vi "S4GUI.vi"() -> ()   [LabVIEW 2018] (continued)
      tunnel: "Input Cluster" -> [_ _ _ _ _ _ _ _ _ _ _ _ _ _ _ _ w2328 w2364 _ _ _ _ _ _ _ _ _ _ _ _ _ _ _ _ _ _ _ _ _ _ _ _ _ _ _ _ _ _ _ _ _ _ _ _ _ _ _ _ _ _ _ _ _ _ _ _ _ _ _ _ _ _ _ _ _ _ _ _ _ _ _ _ _ _ _ _ _ _ _ _ _ _ _ _ _ _ _ _ _ _ _ _ _ _ _ _ _ _ _]
      tunnel: w60 -> [_ _ _ _ _ _ _ _ _ _ _ _ _ _ _ _ _ _ _ _ _ _ w3202 _ _ _ w4393 w4574 w4763 w4947 _ _ w5157 w5348 w5470 w5593 w5719 _ _ _ _ _ _ _ _ _ _ _ _ _ _ _ _ _ _ _ _ _ _ _ _ _ _ _ _ _ _ _ _ _ _ _ _ _ _ _ _ _ _ _ _ _ _ _ _ _ _ _ _ _ _ _ _ _ _ _ _ _ _ _ _ _ _ _ _ _ _ _ _]
      tunnel: w59 -> [_ _ _ _ _ _ _ _ _ _ _ _ _ _ _ _ _ _ _ _ _ _ w3201 _ _ _ _ w4577 w4766 w4950 _ _ w5161 w5347 w5469 w5594 w5718 _ _ _ _ _ _ _ _ _ _ _ _ _ _ _ _ _ _ _ _ _ _ _ _ _ _ _ _ _ _ _ _ _ _ _ _ _ _ _ _ _ _ _ _ _ _ _ _ _ _ _ _ _ _ _ _ _ _ _ _ _ _ _ _ _ _ _ _ _ _ _ _]
      tunnel: "Observer" -> [_ _ _ _ _ _ _ _ _ _ _ _ _ _ _ _ _ _ _ _ _ _ w3200 _ _ _ w4394 w4575 w4764 _ _ _ w5158 w5346 w5468 w5592 w5717 _ _ _ _ _ _ _ _ _ _ _ _ _ _ _ _ _ _ _ _ _ _ _ _ _ _ _ _ _ _ _ _ _ _ _ _ _ _ _ _ _ _ _ _ _ _ _ _ _ _ _ _ _ _ _ _ _ _ _ _ _ _ _ _ _ _ _ _ _ _ _ _]
      event Timeout {
        # "Obtém os valores de status dos\ndispositivos de cada servidor para\napresentar nos indicadores da GUI."
        # "Trata as tarefas individuais de \ncada servidor (ACS1,...,ACS4, \nICS, TCS, SyncBox)"
        # "Determina a sequência de\ntarefas dos servidores\npara uma observação, de \nacordo com o modo de \noperação (disparado com \nos botões START)"
        # "execução dos botões\n no modo sincrono."
        # "execução dos botões\n no modo assincrono."
        # "Instrument States.<device> State\n\n0: nao fez INIT e está parado (mode = IDLE ou WAITING\n                                                    contdition = default)\n1: nao fez INIT e está movendo (mode = IDLE ou WAITING\n                                                    contdition = BUSY)\n\n2: fez INIT e está parado (mode = default)\n                                            condition = READY)\n3: fez INIT e está movendo (mode = default)\n                                            condition = BUSY)"
        n76 = event-data() -> ()  [unwired: 1 in, 2 out]
        n77 = disable-structure shown="Enabled" {
          disable-tunnel: w137 -> [w145 w147]
          disable-tunnel: w136 -> [w144 w146]
          disable-tunnel: [w142 w146] -> w125
          disable-tunnel: [w141 w147] -> w124
          frame Disabled {
            n78 = call "Elapsed Time"() -> ("Time has Elapsed"=w140:bool)  [unwired: 12 in, 7 out]
            n79 = call "Elapsed Time3"() -> ("Time has Elapsed"=w143:bool)  [unwired: 12 in, 7 out]
            n80 = call "Write Status_timeout.vi"("error in (no error)"=w144, "TCS_timeout"=w143, "Status_timeout"=w140, "S4ACS_GUI in"=w145) -> ("error out"=w142:errorcluster, "S4ACS_GUI out"=w141:refnum<class "S4GUI.lvclass">)  [unwired: 6 in]
          }
          frame Enabled {
          }
        }
        n81 = call-dynamic "HandlePauseAsync.vi"("error in (no error)"=w125, "S4GUI in"=w124) -> ("error out"=w121:errorcluster, "S4GUI out"=w123:refnum<class "S4GUI.lvclass">)  [unwired: 8 in]
        n82 = call-dynamic "HandleStopAsync.vi"("error in (no error)"=w121, "S4GUI in"=w123) -> ("error out"=w120:errorcluster, "S4GUI out"=w122:refnum<class "S4GUI.lvclass">)  [unwired: 8 in]
        n83 = call-dynamic "HandleAbortAsync.vi"("error in (no error)"=w120, "S4GUI in"=w122) -> ("error out"=w114:errorcluster, "S4GUI out"=w115:refnum<class "S4GUI.lvclass">)  [unwired: 8 in]
        n84 = call-dynamic "HandlePauseSync.vi"("error in (no error)"=w114, "S4GUI in"=w115) -> ("error out"=w113:errorcluster, "S4GUI out"=w112:refnum<class "S4GUI.lvclass">)  [unwired: 8 in]
        n85 = call-dynamic "HandleStopSync.vi"("error in (no error)"=w113, "S4GUI in"=w112) -> ("error out"=w117:errorcluster, "S4GUI out"=w119:refnum<class "S4GUI.lvclass">)  [unwired: 8 in]
        n86 = call-dynamic "HandleAbortSync.vi"("error in (no error)"=w117, "S4GUI in"=w119) -> ("error out"=w116:errorcluster, "S4GUI out"=w118:refnum<class "S4GUI.lvclass">)  [unwired: 8 in]
        n87 = call-dynamic "HandleObservation.vi"("error in (no error)"=w116, "S4ACS_GUI in"=w118) -> ("error out"=w130:errorcluster, "S4ACS_GUI out"=w131:refnum<class "S4GUI.lvclass">)  [unwired: 8 in]
        n88 = call-dynamic "HandleServers.vi"("error in (no error)"=w130, "S4ACS_GUI in"=w131) -> ("error out"=w139:errorcluster, "S4ACS_GUI out"=w138:refnum<class "S4GUI.lvclass">)  [unwired: 8 in]
        n89 = call-dynamic "GetStatus.vi"("error in (no error)"=w139, "S4ACS_GUI in"=w138) -> ("error out"=w127:errorcluster, "output cluster"=w132:T9, "Cluster Disable"=w129:T10, "S4ACS_GUI out"=w128:refnum<class "S4GUI.lvclass">)  [unwired: 6 in]
        n90 = call "Read cfg file.vi"("error in (no error)"=w127, "S4ACS_GUI in"=w128) -> ("error out"=w109:errorcluster, "cfg file"=w126:string, "S4ACS_GUI out"=w110:refnum<class "S4GUI.lvclass">)  [unwired: 7 in]
        n91 = call "Elapsed Time2"() -> ("Time has Elapsed"=w111:bool)  [unwired: 12 in, 7 out]
        n92 = case shown="True" w111 {
          selector: w111 -> [_ w175]
          tunnel: w132 -> [_ w178]
          tunnel: w129 -> [_ w177]
          tunnel: w126 -> [_ w176]
          tunnel: w110 -> [w149 w172]
          tunnel: w109 -> [w148 w171]
          tunnel: [w149 w169] -> w108
          tunnel: [w148 w166] -> w107
          frame False {
          }
          frame True {
            # "MODE:\nF -> photometric\nT -> polarimetric"
            n93 = stacked-sequence {
              tunnel: w178 -> [w271 w272 w274 w276 w283 w313 w317 w466 w566 w805 _ _ _ _ _ w995 w1155 w1288 w1421]
              tunnel: [_ _ _ _ _ _ _ w464 _ _ _ _ _ _ _ _ _ _ _] -> w150
              tunnel: w177 -> [_ _ _ _ _ _ _ _ _ _ w828 w875 w887 w899 w911 _ _ _ _]
              tunnel: w175 -> [_ _ _ _ _ _ w314 _ w561 _ _ _ _ _ _ _ _ _ _]
              tunnel: w176 -> [_ _ _ _ _ _ _ _ _ _ _ _ _ _ _ w990 _ _ _]
              frame #0 {
                w233 = u32 240 ("Tab Control Pane Dimension:Width")
                w234 = u32 300 ("Tab Control Pane Dimension:Height")
                n94 = Unbundle By Name(w271) -> ("TCSPD_connection"=→"TCSPD":bool, "TCS extended"=w268:string)
                n95 = Match Pattern(string=w268, regular expression="RA=") -> (after substring=w264:string)  [unwired: 1 in, 3 out]
                n96 = Match Pattern(string=w264, regular expression="DEC=") -> (before substring=→"RA":string, after substring=w263:string)  [unwired: 1 in, 2 out]
                n97 = Match Pattern(string=w263, regular expression="EQUINOX=") -> (before substring=→"DEC":string, after substring=w262:string)  [unwired: 1 in, 2 out]
                n98 = Match Pattern(string=w262, regular expression="AIRMASS=") -> (after substring=w258:string)  [unwired: 1 in, 3 out]
                n99 = Match Pattern(string=w258, regular expression="TCSHA=") -> (before substring=→"Air Mass":string, after substring=w257:string)  [unwired: 1 in, 2 out]
                n100 = Match Pattern(string=w257, regular expression="TCSDATE=") -> (before substring=→"Hour Angle":string, after substring=w255:string)  [unwired: 1 in, 2 out]
                n101 = Match Pattern(string=w255, regular expression="TELFOCUS=") -> (before substring=→"Date":string, after substring=w251:string)  [unwired: 1 in, 2 out]
                n102 = Match Pattern(string=w251, regular expression="EXTTEMP=") -> (before substring=→"Telescope Focus":string, after substring=w250:string)  [unwired: 1 in, 2 out]
                n103 = Match Pattern(string=w250, regular expression="PRESSURE=") -> (before substring=→"Outside Temp":string, after substring=w249:string)  [unwired: 1 in, 2 out]
                n104 = property on="Tab CH2" class="TabCtl (strict)"("PaneHeight"=w234, "PaneWidth"=w233) -> ()  [unwired: 2 in, 2 out]
                n105 = property on="Tab CH1" class="TabCtl (strict)"("PaneHeight"=w234, "PaneWidth"=w233) -> ()  [unwired: 2 in, 2 out]
                n106 = property on="Tab CH3" class="TabCtl (strict)"("PaneHeight"=w234, "PaneWidth"=w233) -> ()  [unwired: 2 in, 2 out]
                n107 = Match Pattern(string=w249, regular expression="HUMIDITY=") -> (before substring=→"Pressure":string, after substring=w238:string)  [unwired: 1 in, 2 out]
                n108 = property on="Tab CH4" class="TabCtl (strict)"("PaneHeight"=w234, "PaneWidth"=w233) -> ()  [unwired: 2 in, 2 out]
                n109 = Match Pattern(string=w238, regular expression="JD=") -> (before substring=→"Humidity":string, after substring=w239:string)  [unwired: 1 in, 2 out]
                n110 = Match Pattern(string=w239, regular expression="SD=") -> (before substring=→"Julian Date":string, after substring=→"Sideral Time":string)  [unwired: 1 in, 2 out]
              }
              frame #1 {
                n111 = Unbundle By Name(w272) -> ()  [unwired: 1 out]
              }
              frame #2 {
                n112 = Unbundle By Name(w274) -> ("Trigger Mode Status"=→"String":string)
              }
              frame #3 {
                n113 = Unbundle By Name(w276) -> ("Trigger General Status"=→"String 2":string)
              }
              frame #4 {
                n114 = Unbundle By Name(w283) -> ("Instrument Status"=w282:T11, "Instrument States.WPROT State"=w281:i32, "Instrument Pos Names.WPROT posname"=w280:string, "Instrument Pos Names.WPSEL posname"=w279:string, "Instrument Pos Names.CALW posname"=w278:string, "Instrument Pos Names.ASEL posname"=w277:string)
                n115 = stacked-sequence {
                  tunnel: w282 -> [w290 w293 w296 w298 w300 w303 w306 w308 w310]
                  tunnel: w281 -> [w286 _ _ _ _ _ _ _ _]
                  tunnel: w280 -> [_ w291 _ _ _ _ _ _ _]
                  tunnel: w279 -> [_ _ w294 _ _ _ _ _ _]
                  tunnel: w278 -> [_ _ _ _ _ w301 _ _ _]
                  tunnel: w277 -> [_ _ _ _ _ _ w304 _ _]
                  frame #0 {
                    # "Pisca quando BUSY"
                    n116 = Unbundle By Name(w290) -> ("WPROT pos"=w287:dbl)
                    "WaveplatePos 2" <- w287
                    n117 = Equal?(x=w286, y=3) -> (x = y?=w284:bool)
                    n118 = property on="WaveplatePos 2" class="DigNum (strict)"("Blinking"=w284) -> ()  [unwired: 2 in, 2 out]
                    n119 = Number To Fractional String(number=w287, precision (6)=i16 1) -> (F-format string=→"Angle":string)  [unwired: 2 in]
                  }
                  frame #1 {
                    n120 = Unbundle By Name(w293) -> ("WPROT pos"=→"Position WPROT":dbl)
                    "PosName WPROT" <- w291
                  }
                  frame #2 {
                    n121 = Unbundle By Name(w296) -> ("WPSEL pos"=→"Position WPSEL":dbl)
                    "PosName WPSEL" <- w294
                  }
                  frame #3 {
                    n122 = Unbundle By Name(w298) -> ("GMIR pos"=→"Position GMIR":dbl)
                  }
                  frame #4 {
                    n123 = Unbundle By Name(w300) -> ("GFOC pos"=→"Position GFOC":dbl)
                  }
                  frame #5 {
                    n124 = Unbundle By Name(w303) -> ("CALW pos"=→"Position CALW":dbl)
                    "PosName CALW" <- w301
                  }
                  frame #6 {
                    n125 = Unbundle By Name(w306) -> ("ASEL pos"=→"PosName ASEL":dbl)
                    "PosName ASEL" <- w304
                  }
                  frame #7 {
                    n126 = Unbundle By Name(w308) -> ("connection"=→"S4ICSoft":bool)
                  }
                  frame #8 {
                    n127 = Unbundle By Name(w310) -> ("String Status"=→"Status":string)
                  }
                }
              }
              frame #5 {
                n128 = Unbundle By Name(w313) -> ("Sync Box State"=→"Current State":i32, "Trigger_connection"=→"Sync Box" →"LedExtSync":bool)
              }
              frame #6 {
                n129 = Unbundle By Name(w317) -> ("Instrument States"=w316:T12, "Instrument Pos Names"=w315:T13)
                n130 = stacked-sequence {
                  tunnel: w316 -> [w326 w352 w371 w410 w439 w453]
                  tunnel: w315 -> [w322 _ w369 w406 _ _]
                  tunnel: w314 -> [w320 _ w363 w403 _ _]
                  frame #0 {
                    # "WPSEL"
                    n131 = Unbundle By Name(w322) -> ("WPSEL posname"=w318:string)
                    n132 = Unbundle By Name(w326) -> ("WPSEL State"=w325:i32)
                    n133 = local read "WPSEL Status"() -> (w321:bool)
                    n134 = case shown="2" w325 {
                      tunnel: [cluster{u32, u32}[] [{9868950, 9868950}, {9868950, 9868950}] ("Colors [4]") cluster{u32, u32}[] [{9868950, 9868950}, {9868950, 9868950}] ("Colors [4]") cluster{u32, u32}[] [{16318208, 16318208}, {16318208, 16318208}] ("Colors [4]") cluster{u32, u32}[] [{6618880, 2424594}, {6618880, 2424594}] ("Colors [4]") w341] -> w324
                      tunnel: [FALSE ("WPROT Status") FALSE ("WPROT Status") TRUE ("WPROT Status") FALSE ("WPROT Status") w343] -> w323
                      tunnel: w321 -> [_ _ _ _ w342]
                      tunnel: w320 -> [_ _ _ _ w340]
                      tunnel: ["" "" "" w336 ""] -> w319
                      tunnel: w318 -> [_ _ _ w336 _]
                      frame Default {
                      }
                      frame 0 {
                      }
                      frame 1 {
                      }
                      frame 2 {
                      }
                      frame 3 {
                        n135 = case shown="True" w342 {
                          tunnel: [cluster{u32, u32}[] [{7563008, 7563008}, {7563008, 7563008}] ("Colors [4]") cluster{u32, u32}[] [{16318208, 16318208}, {16318208, 16318208}] ("Colors [4]")] -> w341
                          frame False {
                          }
                          frame True {
                          }
                        }
                        n136 = case shown="True" w340 {
                          tunnel: [w344 w346] -> w343
                          tunnel: w342 -> [w344 w345]
                          frame False {
                          }
                          frame True {
                            n137 = Not(x=w345) -> (.not. x?=w346:bool)
                          }
                        }
                      }
                    }
                    "WPSEL Status" <- w323
                    "Waveplate" <- w323
                    n138 = property on="Waveplate" class="Bool (strict)"("Colors [4]"=w324, "BoolText.Text"=w319) -> ()  [unwired: 2 in, 2 out]
                    n139 = property on="WPSEL Status" class="Bool (strict)"("Colors [4]"=w324) -> ()  [unwired: 2 in, 2 out]
                  }
                  frame #1 {
                    # "WPROT"
                    n140 = Unbundle By Name(w352) -> ("WPROT State"=w351:i32)
                    n141 = case shown="2" w351 {
                      tunnel: [cluster{u32, u32}[] [{9868950, 9868950}, {9868950, 9868950}] ("Colors [4]") cluster{u32, u32}[] [{9868950, 9868950}, {9868950, 9868950}] ("Colors [4]") cluster{u32, u32}[] [{16318208, 16318208}, {16318208, 16318208}] ("Colors [4]") cluster{u32, u32}[] [{6618880, 6618880}, {6618880, 6618880}] ("Colors [4]") cluster{u32, u32}[] [{16318208, 16318208}, {16318208, 16318208}] ("Colors [4]")] -> w350
                      tunnel: [FALSE ("WPROT Status") FALSE ("WPROT Status") TRUE ("WPROT Status") FALSE ("WPROT Status") TRUE ("WPROT Status")] -> w349
                      frame Default {
                      }
                      frame 0 {
                      }
                      frame 1 {
                      }
                      frame 2 {
                      }
                      frame 3 {
                      }
                    }
                    "WPROT Status" <- w349
                    n142 = property on="WPROT Status" class="Bool (strict)"("Colors [4]"=w350) -> ()  [unwired: 2 in, 2 out]
                  }
                  frame #2 {
                    # "CALW"
                    n143 = Unbundle By Name(w371) -> ("CALW State"=w370:i32)
                    n144 = Unbundle By Name(w369) -> ("CALW posname"=w368:string)
                    n145 = local read "CALW Status"() -> (w364:bool)
                    n146 = case shown="Default" w370 {
                      tunnel: [cluster{u32, u32}[] [{9868950, 9868950}, {9868950, 9868950}] ("Colors [4]") cluster{u32, u32}[] [{9868950, 9868950}, {9868950, 9868950}] ("Colors [4]") cluster{u32, u32}[] [{16318208, 16318208}, {16318208, 16318208}] ("Colors [4]") cluster{u32, u32}[] [{6618880, 6618880}, {6618880, 6618880}] ("Colors [4]") w392] -> w365
                      tunnel: [FALSE ("WPROT Status") FALSE ("WPROT Status") TRUE ("WPROT Status") FALSE ("WPROT Status") w394] -> w367
                      tunnel: w368 -> [_ _ _ w382 _]
                      tunnel: ["" "" "" w381 ""] -> w366
                      tunnel: w364 -> [_ _ _ _ w393]
                      tunnel: w363 -> [_ _ _ _ w391]
                      frame Default {
                      }
                      frame 0 {
                      }
                      frame 1 {
                      }
                      frame 2 {
                        n147 = case shown="\"SHUTTER\"" w382 {
                          tunnel: ["" "DEPOL" "POL" "OFF" "PIN" "SHT"] -> w381
                          frame Default {
                          }
                          frame "DEPOLARIZER" {
                          }
                          frame "POLARIZER" {
                          }
                          frame "OFF" {
                          }
                          frame "PINHOLE" {
                          }
                          frame "SHUTTER" {
                          }
                        }
                      }
                      frame 3 {
                        n148 = case shown="False" w393 {
                          tunnel: [cluster{u32, u32}[] [{7563008, 7563008}, {7563008, 7563008}] ("Colors [4]") cluster{u32, u32}[] [{16318208, 16318208}, {16318208, 16318208}] ("Colors [4]")] -> w392
                          frame False {
                          }
                          frame True {
                          }
                        }
                        n149 = case shown="True" w391 {
                          tunnel: [w396 w398] -> w394
                          tunnel: w393 -> [w396 w397]
                          frame False {
                          }
                          frame True {
                            n150 = Not(x=w397) -> (.not. x?=w398:bool)
                          }
                        }
                      }
                    }
                    "CALW Status" <- w367
                    "PCS" <- w367
                    n151 = property on="CALW Status" class="Bool (strict)"("Colors [4]"=w365) -> ()  [unwired: 2 in, 2 out]
                    n152 = property on="PCS" class="Bool (strict)"("Colors [4]"=w365, "BoolText.Text"=w366) -> ()  [unwired: 2 in, 2 out]
                  }
                  frame #3 {
                    # "ASEL"
                    n153 = Unbundle By Name(w410) -> ("ASEL State"=w409:i32)
                    n154 = Unbundle By Name(w406) -> ("ASEL posname"=w402:string)
                    n155 = local read "ASEL Status"() -> (w404:bool)
                    n156 = case shown="Default" w402 {
                      selector: w402 -> [w411 _ _]
                      tunnel: [w411 "OFF" ("y") "ON" ("y")] -> w401
                      frame Default {
                      }
                      frame "OFF" {
                      }
                      frame "ON" {
                      }
                    }
                    n157 = case shown="2" w409 {
                      tunnel: [cluster{u32, u32}[] [{9868950, 9868950}, {9868950, 9868950}] ("Colors [4]") cluster{u32, u32}[] [{9868950, 9868950}, {9868950, 9868950}] ("Colors [4]") cluster{u32, u32}[] [{16318208, 16318208}, {16318208, 16318208}] ("Colors [4]") cluster{u32, u32}[] [{6618880, 6618880}, {6618880, 6618880}] ("Colors [4]") w430] -> w407
                      tunnel: [FALSE ("WPROT Status") FALSE ("WPROT Status") TRUE FALSE ("WPROT Status") w429] -> w408
                      tunnel: w401 -> [_ _ _ w424 _]
                      tunnel: ["" ("y") "" ("y") "" ("y") w424 "" ("y")] -> w405
                      tunnel: w404 -> [_ _ _ _ w427]
                      tunnel: w403 -> [_ _ _ _ w426]
                      frame Default {
                      }
                      frame 0 {
                      }
                      frame 1 {
                      }
                      frame 2 {
                      }
                      frame 3 {
                        n158 = case shown="True" w427 {
                          tunnel: [cluster{u32, u32}[] [{7563008, 7563008}, {7563008, 7563008}] ("Colors [4]") cluster{u32, u32}[] [{16318208, 16318208}, {16318208, 16318208}] ("Colors [4]")] -> w430
                          frame False {
                          }
                          frame True {
                          }
                        }
                        n159 = case shown="True" w426 {
                          tunnel: [w431 w433] -> w429
                          tunnel: w427 -> [w431 w432]
                          frame False {
                          }
                          frame True {
                            n160 = Not(x=w432) -> (.not. x?=w433:bool)
                          }
                        }
                      }
                    }
                    "ASEL Status" <- w408
                    "Analyzer" <- w408
                    n161 = property on="Analyzer" class="Bool (strict)"("Colors [4]"=w407, "BoolText.Text"=w405) -> ()  [unwired: 2 in, 2 out]
                    n162 = property on="ASEL Status" class="Bool (strict)"("Colors [4]"=w407) -> ()  [unwired: 2 in, 2 out]
                  }
                  frame #4 {
                    # "GMIR"
                    n163 = Unbundle By Name(w439) -> ("GMIR State"=w438:i32)
                    n164 = case shown="2" w438 {
                      tunnel: [cluster{u32, u32}[] [{9868950, 9868950}, {9868950, 9868950}] ("Colors [4]") cluster{u32, u32}[] [{9868950, 9868950}, {9868950, 9868950}] ("Colors [4]") cluster{u32, u32}[] [{16318208, 16318208}, {16318208, 16318208}] ("Colors [4]") cluster{u32, u32}[] [{6618880, 6618880}, {6618880, 6618880}] ("Colors [4]") cluster{u32, u32}[] [{16318208, 16318208}, {16318208, 16318208}] ("Colors [4]")] -> w437
                      tunnel: [FALSE ("WPROT Status") FALSE ("WPROT Status") TRUE ("WPROT Status") FALSE ("WPROT Status") TRUE ("WPROT Status")] -> w436
                      frame Default {
                      }
                      frame 0 {
                      }
                      frame 1 {
                      }
                      frame 2 {
                      }
                      frame 3 {
                      }
                    }
                    "GMIR Status" <- w436
                    n165 = property on="GMIR Status" class="Bool (strict)"("Colors [4]"=w437) -> ()  [unwired: 2 in, 2 out]
                  }
                  frame #5 {
                    # "GFOC"
                    n166 = Unbundle By Name(w453) -> ("GFOC State"=w452:i32)
                    n167 = case shown="0" w452 {
                      tunnel: [cluster{u32, u32}[] [{9868950, 9868950}, {9868950, 9868950}] ("Colors [4]") cluster{u32, u32}[] [{9868950, 9868950}, {9868950, 9868950}] ("Colors [4]") cluster{u32, u32}[] [{16318208, 16318208}, {16318208, 16318208}] ("Colors [4]") cluster{u32, u32}[] [{6618880, 6618880}, {6618880, 6618880}] ("Colors [4]") cluster{u32, u32}[] [{16318208, 16318208}, {16318208, 16318208}] ("Colors [4]")] -> w451
                      tunnel: [FALSE ("WPROT Status") FALSE ("WPROT Status") TRUE ("WPROT Status") FALSE ("WPROT Status") TRUE ("WPROT Status")] -> w450
                      frame Default {
                      }
                      frame 0 {
                      }
                      frame 1 {
                      }
                      frame 2 {
                      }
                      frame 3 {
                      }
                    }
                    "GFOC Status" <- w450
                    n168 = property on="GFOC Status" class="Bool (strict)"("Colors [4]"=w451) -> ()  [unwired: 2 in, 2 out]
                  }
                }
              }
              frame #7 {
                n169 = Unbundle By Name(w466) -> ("Instrument Pos Names"=w465:T13)
                n170 = stacked-sequence {
                  tunnel: w465 -> [w468 w485 w510 w536]
                  tunnel: [_ _ _ w537] -> w464
                  frame #0 {
                    n171 = Unbundle By Name(w468) -> ("WPSEL posname"=w467:string)
                    n172 = case shown="\"L/2\", \"L/4\", \"OFF\"" w467 {
                      selector: w467 -> [_ w469]
                      frame "False", Default {
                      }
                      frame "L/2", "L/4", "OFF" {
                        n173 = First Call?() -> (First Call?: T/F=w470:bool)
                        n174 = case shown="True" w470 {
                          tunnel: w469 -> [_ w471]
                          frame False {
                          }
                          frame True {
                            n175 = case shown="\"L/2\"" w471 {
                              frame "False", Default {
                              }
                              frame "L/2" {
                                w472 = u16 1 items=["OFF", "Lambda/2", "Lambda/4"] ("Lambda Selector")
                                n176 = property on="Lambda Selector" class="Ring (strict)"(error in=errorcluster {"status"=FALSE, "code"=0, "source"=""} ("error in (no error)"), "Value"=w472) -> (error out=w474:errorcluster)  [unwired: 1 in, 1 out]
                                n177 = property on="Lambda Selector" class="Ring (strict)"(error in=w474, "RingText.Text"="Lambda/2" ("Boolean Text.Text")) -> ()  [unwired: 1 in, 2 out]
                              }
                              frame "L/4" {
                                w476 = u16 2 items=["OFF", "Lambda/2", "Lambda/4"] ("Lambda Selector")
                                n178 = property on="Lambda Selector" class="Ring (strict)"(error in=errorcluster {"status"=FALSE, "code"=0, "source"=""} ("error in (no error)"), "Value"=w476) -> (error out=w478:errorcluster)  [unwired: 1 in, 1 out]
                                n179 = property on="Lambda Selector" class="Ring (strict)"(error in=w478, "RingText.Text"="Lambda/4" ("Boolean Text.Text")) -> ()  [unwired: 1 in, 2 out]
                              }
                              frame "OFF" {
                                w480 = u16 0 items=["OFF", "Lambda/2", "Lambda/4"] ("Lambda Selector")
                                n180 = property on="Lambda Selector" class="Ring (strict)"(error in=errorcluster {"status"=FALSE, "code"=0, "source"=""} ("error in (no error)"), "Value"=w480) -> (error out=w482:errorcluster)  [unwired: 1 in, 1 out]
                                n181 = property on="Lambda Selector" class="Ring (strict)"(error in=w482, "RingText.Text"="OFF" ("Boolean Text.Text")) -> ()  [unwired: 1 in, 2 out]
                              }
                            }
                          }
                        }
                      }
                    }
                  }
                  frame #1 {
                    n182 = Unbundle By Name(w485) -> ("CALW posname"=w484:string)
                    n183 = case shown="\"DEPOLARIZER\", \"OFF\", \"PINHOLE\", \"POLARIZER\", \"SHUTTER\"" w484 {
                      selector: w484 -> [_ w486]
                      frame "False", Default {
                      }
                      frame "DEPOLARIZER", "OFF", "PINHOLE", "POLARIZER", "SHUTTER" {
                        n184 = First Call?() -> (First Call?: T/F=w487:bool)
                        n185 = case shown="True" w487 {
                          tunnel: w486 -> [_ w488]
                          frame False {
                          }
                          frame True {
                            n186 = case shown="\"OFF\"" w488 {
                              frame "False", Default {
                              }
                              frame "POLARIZER" {
                                w489 = u16 1 items=["OFF", "POLARIZER", "PINHOLE", "SHUTTER", "DEPOLARIZER"] ("Calibrator Selector")
                                n187 = property on="Calibrator Selector" class="Ring (strict)"(error in=errorcluster {"status"=FALSE, "code"=0, "source"=""} ("error in (no error)"), "Value"=w489) -> (error out=w491:errorcluster)  [unwired: 1 in, 1 out]
                                n188 = property on="Calibrator Selector" class="Ring (strict)"(error in=w491, "RingText.Text"="POLARIZER" ("Boolean Text.Text")) -> ()  [unwired: 1 in, 2 out]
                              }
                              frame "DEPOLARIZER" {
                                w493 = u16 4 items=["OFF", "POLARIZER", "PINHOLE", "SHUTTER", "DEPOLARIZER"] ("Calibrator Selector")
                                n189 = property on="Calibrator Selector" class="Ring (strict)"(error in=errorcluster {"status"=FALSE, "code"=0, "source"=""} ("error in (no error)"), "Value"=w493) -> (error out=w495:errorcluster)  [unwired: 1 in, 1 out]
                                n190 = property on="Calibrator Selector" class="Ring (strict)"(error in=w495, "RingText.Text"="DEPOLARIZER" ("Boolean Text.Text")) -> ()  [unwired: 1 in, 2 out]
                              }
                              frame "PINHOLE" {
                                w497 = u16 2 items=["OFF", "POLARIZER", "PINHOLE", "SHUTTER", "DEPOLARIZER"] ("Calibrator Selector")
                                n191 = property on="Calibrator Selector" class="Ring (strict)"(error in=errorcluster {"status"=FALSE, "code"=0, "source"=""} ("error in (no error)"), "Value"=w497) -> (error out=w499:errorcluster)  [unwired: 1 in, 1 out]
                                n192 = property on="Calibrator Selector" class="Ring (strict)"(error in=w499, "RingText.Text"="PINHOLE" ("Boolean Text.Text")) -> ()  [unwired: 1 in, 2 out]
                              }
                              frame "SHUTTER" {
                                w501 = u16 3 items=["OFF", "POLARIZER", "PINHOLE", "SHUTTER", "DEPOLARIZER"] ("Calibrator Selector")
                                n193 = property on="Calibrator Selector" class="Ring (strict)"(error in=errorcluster {"status"=FALSE, "code"=0, "source"=""} ("error in (no error)"), "Value"=w501) -> (error out=w503:errorcluster)  [unwired: 1 in, 1 out]
                                n194 = property on="Calibrator Selector" class="Ring (strict)"(error in=w503, "RingText.Text"="SHUTTER" ("Boolean Text.Text")) -> ()  [unwired: 1 in, 2 out]
                              }
                              frame "OFF" {
                                w505 = u16 0 items=["OFF", "POLARIZER", "PINHOLE", "SHUTTER", "DEPOLARIZER"] ("Calibrator Selector")
                                n195 = property on="Calibrator Selector" class="Ring (strict)"(error in=errorcluster {"status"=FALSE, "code"=0, "source"=""} ("error in (no error)"), "Value"=w505) -> (error out=w507:errorcluster)  [unwired: 1 in, 1 out]
                                n196 = property on="Calibrator Selector" class="Ring (strict)"(error in=w507, "RingText.Text"="OFF" ("Boolean Text.Text")) -> ()  [unwired: 1 in, 2 out]
                              }
                            }
                          }
                        }
                      }
                    }
                  }
                  frame #2 {
                    n197 = Unbundle By Name(w510) -> ("WPROT posname"=w509:string)
                    "Name" <- w509
                    n198 = stacked-sequence {
                      tunnel: w509 -> [_ w512]
                      frame #0 {
                        w511 = FALSE
                        "ledP0" <- w511
                        "ledP1" <- w511
                        "ledP2" <- w511
                        "ledP3" <- w511
                        "ledP4" <- w511
                        "ledP5" <- w511
                        "ledP6" <- w511
                        "ledP7" <- w511
                        "ledP8" <- w511
                        "ledP9" <- w511
                        "ledP10" <- w511
                        "ledP11" <- w511
                        "ledP12" <- w511
                        "ledP13" <- w511
                        "ledP14" <- w511
                        "ledP15" <- w511
                      }
                      frame #1 {
                        n199 = case shown="\"WP15\"" w512 {
                          frame Default {
                          }
                          frame "WP1" {
                            n200 = local write "ledP0"(TRUE ("ledP0")) -> ()
                          }
                          frame "WP2" {
                            n201 = local write "ledP1"(TRUE ("ledP0")) -> ()
                          }
                          frame "WP3" {
                            n202 = local write "ledP2"(TRUE ("ledP0")) -> ()
                          }
                          frame "WP4" {
                            n203 = local write "ledP3"(TRUE ("ledP0")) -> ()
                          }
                          frame "WP5" {
                            n204 = local write "ledP4"(TRUE ("ledP0")) -> ()
                          }
                          frame "WP6" {
                            n205 = local write "ledP5"(TRUE ("ledP0")) -> ()
                          }
                          frame "WP7" {
                            n206 = local write "ledP6"(TRUE ("ledP0")) -> ()
                          }
                          frame "WP8" {
                            n207 = local write "ledP7"(TRUE ("ledP0")) -> ()
                          }
                          frame "WP9" {
                            n208 = local write "ledP8"(TRUE ("ledP0")) -> ()
                          }
                          frame "WP10" {
                            n209 = local write "ledP9"(TRUE ("ledP0")) -> ()
                          }
                          frame "WP11" {
                            n210 = local write "ledP10"(TRUE ("ledP0")) -> ()
                          }
                          frame "WP12" {
                            n211 = local write "ledP11"(TRUE ("ledP0")) -> ()
                          }
                          frame "WP13" {
                            n212 = local write "ledP12"(TRUE ("ledP0")) -> ()
                          }
                          frame "WP14" {
                            n213 = local write "ledP13"(TRUE ("ledP0")) -> ()
                          }
                          frame "WP15" {
                            n214 = local write "ledP14"(TRUE ("ledP0")) -> ()
                          }
                          frame "WP16" {
                            n215 = local write "ledP15"(TRUE ("ledP0")) -> ()
                          }
                        }
                      }
                    }
                  }
                  frame #3 {
                    w540 = "OFF" ("Boolean Text.Text")
                    # "Polarimetria:   ASEL = ON  &   (WPSEL =L/2 or L/4)\n\nFotometria:    ASEL=OFF & WPSEL = OFF & CALW = OFF"
                    n216 = Unbundle By Name(w536) -> ("ASEL posname"=w531:string, "WPSEL posname"=w533:string, "ASEL posname"=w532:string)
                    n217 = Unbundle By Name(w536) -> ("WPSEL posname"=w543:string, "CALW posname"=w544:string, "ASEL posname"=w538:string)
                    n218 = Equal?(x=w531, y="ON" ("Boolean Text.Text")) -> (x = y?=w534:bool)
                    n219 = case shown="True" w534 {
                      tunnel: w533 -> [w553 w558]
                      tunnel: w532 -> [w552 _]
                      tunnel: w531 -> [w549 _]
                      tunnel: [FALSE ("Polarimetric Mode") w555] -> w530
                      tunnel: [w545 FALSE ("Photometric Mode")] -> w529
                      frame False {
                        w548 = "OFF" ("Boolean Text.Text")
                        n220 = Equal?(x=w549, y=w548) -> (x = y?=w547:bool)
                        n221 = Equal?(x=w552, y=w548) -> (x = y?=w550:bool)
                        n222 = Equal?(x=w553, y=w548) -> (x = y?=w551:bool)
                        n223 = Compound Arithmetic op=AND(w547, w551, w550) -> (w545:bool)
                      }
                      frame True {
                        n224 = Equal?(x="L/2" ("Boolean Text.Text"), y=w558) -> (x = y?=w559:bool)
                        n225 = Equal?(x="L/4" ("Boolean Text.Text"), y=w558) -> (x = y?=w556:bool)
                        n226 = Or(x=w559, y=w556) -> (x .or. y?=w555:bool)
                      }
                    }
                    "Polarimetric Mode" <- w530
                    "Photometric Mode" <- w529
                    n227 = Equal?(x=w540, y=w543) -> (x = y?=w541:bool)
                    n228 = Equal?(x=w540, y=w544) -> (x = y?=w542:bool)
                    n229 = Equal?(x=w540, y=w538) -> (x = y?=w539:bool)
                    n230 = Compound Arithmetic op=AND(w541, w542, w539) -> (invert w537:bool)
                  }
                }
              }
              frame #8 {
                n231 = Unbundle By Name(w566) -> ("ChannelA_Status"=w565:T14, "ChannelB_Status"=w564:T14, "ChannelC_Status"=w562:T14, "ChannelD_Status"=w563:T14)
                n232 = stacked-sequence {
                  tunnel: w565 -> [w614 w662 w715 w791 _ _ _]
                  tunnel: w564 -> [w613 w660 w714 _ w794 _ _]
                  tunnel: w563 -> [w611 w657 w712 _ _ _ w802]
                  tunnel: w562 -> [w612 w658 w713 _ _ w798 _]
                  tunnel: w561 -> [_ _ w704 _ _ _ _]
                  frame #0 {
                    n233 = Unbundle By Name(w611) -> ("connection"=w587:bool, "Current exp"=→"Exposure Time ch4":dbl, "Cooler ON/OFF"=w601:i16, "Currently temperature"=w598:i16, "Temperature Status"=w595:string, "target  temp"=w583:i16)
                    n234 = Unbundle By Name(w613) -> ("connection"=w589:bool, "Current exp"=→"Exposure Time ch2":dbl, "Cooler ON/OFF"=w603:i16, "Currently temperature"=w600:i16, "Temperature Status"=w597:string, "target  temp"=w585:i16)
                    n235 = Unbundle By Name(w614) -> ("connection"=w590:bool, "Current exp"=→"Exposure Time ch1":dbl, "Cooler ON/OFF"=w606:i16, "Currently temperature"=w604:i16, "Temperature Status"=w605:string, "target  temp"=w586:i16)
                    n236 = Unbundle By Name(w612) -> ("connection"=w588:bool, "Current exp"=→"Exposure Time ch3":dbl, "Cooler ON/OFF"=w602:i16, "Currently temperature"=w599:i16, "Temperature Status"=w596:string, "target  temp"=w584:i16)
                    n237 = Not Equal To 0?(x=w603) -> (x != 0?=w594:bool)
                    n238 = Not Equal To 0?(x=w601) -> (x != 0?=w592:bool)
                    n239 = First Call?() -> (First Call?: T/F=w581:bool)
                    n240 = First Call?() -> (First Call?: T/F=w582:bool)
                    n241 = First Call?() -> (First Call?: T/F=w580:bool)
                    n242 = Not Equal To 0?(x=w606) -> (x != 0?=w593:bool)
                    n243 = First Call?() -> (First Call?: T/F=w579:bool)
                    n244 = Not Equal To 0?(x=w602) -> (x != 0?=w591:bool)
                    n245 = case shown="True" w581 {
                      tunnel: w585 -> [_ w617]
                      frame False {
                      }
                      frame True {
                        n246 = property on="Target Temp 2" class="DigNum (strict)"("Value"=w617) -> ()  [unwired: 2 in, 2 out]
                      }
                    }
                    n247 = case shown="True" w580 {
                      tunnel: w584 -> [_ w616]
                      frame False {
                      }
                      frame True {
                        n248 = property on="Target Temp 3" class="DigNum (strict)"("Value"=w616) -> ()  [unwired: 2 in, 2 out]
                      }
                    }
                    n249 = case shown="True" w582 {
                      tunnel: w586 -> [_ w618]
                      frame False {
                      }
                      frame True {
                        n250 = property on="Target Temp 1" class="DigNum (strict)"("Value"=w618) -> ()  [unwired: 2 in, 2 out]
                      }
                    }
                    n251 = case shown="True" w579 {
                      tunnel: w583 -> [_ w615]
                      frame False {
                      }
                      frame True {
                        n252 = property on="Target Temp 4" class="DigNum (strict)"("Value"=w615) -> ()  [unwired: 2 in, 2 out]
                      }
                    }
                    n253 = case shown="False" w590 {
                      tunnel: w605 -> [_ w640]
                      tunnel: w604 -> [_ w641]
                      tunnel: w593 -> [_ w642]
                      tunnel: [FALSE w642] -> w578
                      tunnel: [i16 0 ("Currently temperature") w641] -> w577
                      tunnel: ["" ("Temperature Status") w640] -> w576
                      frame False {
                      }
                      frame True {
                      }
                    }
                    "Cooler status 1" <- w578
                    "Curr Temp 1" <- w577
                    "Temp Status 1" <- w576
                    "Panel Temp" <- w577
                    "Cooler" <- w578
                    n254 = case shown="False" w589 {
                      tunnel: w600 -> [_ w635]
                      tunnel: w597 -> [_ w634]
                      tunnel: w594 -> [_ w636]
                      tunnel: [FALSE w636] -> w575
                      tunnel: [i16 0 ("Currently temperature") w635] -> w574
                      tunnel: ["" ("Temperature Status") w634] -> w573
                      frame False {
                      }
                      frame True {
                      }
                    }
                    "Panel Temp 2" <- w574
                    "Curr Temp 2" <- w574
                    "Cooler status 2" <- w575
                    "Panel cooler 2" <- w575
                    "Temp Status 2" <- w573
                    n255 = case shown="False" w587 {
                      tunnel: w598 -> [_ w623]
                      tunnel: w595 -> [_ w622]
                      tunnel: w592 -> [_ w624]
                      tunnel: [FALSE w624] -> w569
                      tunnel: [i16 0 ("Currently temperature") w623] -> w568
                      tunnel: ["" ("Temperature Status") w622] -> w567
                      frame False {
                      }
                      frame True {
                      }
                    }
                    "Cooler status 4" <- w569
                    "Panel Temp 4" <- w568
                    "Curr Temp 4" <- w568
                    "Temp Status 4" <- w567
                    "Panel cooler 4" <- w569
                    n256 = case shown="False" w588 {
                      tunnel: w599 -> [_ w629]
                      tunnel: w596 -> [_ w628]
                      tunnel: w591 -> [_ w630]
                      tunnel: [FALSE w630] -> w572
                      tunnel: [i16 0 ("Currently temperature") w629] -> w571
                      tunnel: ["" ("Temperature Status") w628] -> w570
                      frame False {
                      }
                      frame True {
                      }
                    }
                    "Cooler status 3" <- w572
                    "Panel Temp 3" <- w571
                    "Curr Temp 3" <- w571
                    "Temp Status 3" <- w570
                    "Panel cooler 3" <- w572
                  }
                  frame #1 {
                    n257 = Unbundle By Name(w657) -> ("LastFileImage"=→"Last Image ch4":string, "Temperature Status"=w645:string)
                    n258 = Unbundle By Name(w658) -> ("LastFileImage"=→"Last Image ch3":string, "Temperature Status"=w646:string)
                    n259 = Unbundle By Name(w660) -> ("LastFileImage"=→"Last Image ch2":string, "Temperature Status"=w649:string)
                    n260 = Unbundle By Name(w662) -> ("LastFileImage"=→"Last Image ch1":string, "Temperature Status"=w654:string)
                    n261 = case shown="\"TEMPERATURE_NOT_REACHED\"" w654 {
                      tunnel: [cluster{u32, u32}[] [{6124107, 6124107}, {6124107, 6124107}] ("Colors [4]") cluster{u32, u32}[] [{6618880, 6618880}, {6618880, 6618880}] ("Colors [4]") cluster{u32, u32}[] [{16318208, 16318208}, {16318208, 16318208}] ("Colors [4]") cluster{u32, u32}[] [{8554752, 8554752}, {8554752, 8554752}] ("Colors [4]")] -> w653
                      tunnel: [FALSE FALSE FALSE TRUE] -> w652
                      frame Default {
                      }
                      frame "TEMPERATURE_STABILIZED" {
                      }
                      frame "TEMPERATURE_NOT_STABILIZED" {
                      }
                      frame "TEMPERATURE_NOT_REACHED" {
                      }
                    }
                    n262 = case shown="\"TEMPERATURE_NOT_REACHED\"" w649 {
                      tunnel: [cluster{u32, u32}[] [{6124107, 6124107}, {6124107, 6124107}] ("Colors [4]") cluster{u32, u32}[] [{6618880, 6618880}, {6618880, 6618880}] ("Colors [4]") cluster{u32, u32}[] [{16318208, 16318208}, {16318208, 16318208}] ("Colors [4]") cluster{u32, u32}[] [{8554752, 8554752}, {8554752, 8554752}] ("Colors [4]")] -> w651
                      tunnel: [FALSE FALSE FALSE TRUE] -> w650
                      frame Default {
                      }
                      frame "TEMPERATURE_STABILIZED" {
                      }
                      frame "TEMPERATURE_NOT_STABILIZED" {
                      }
                      frame "TEMPERATURE_NOT_REACHED" {
                      }
                    }
                    n263 = case shown="\"TEMPERATURE_NOT_REACHED\"" w646 {
                      tunnel: [cluster{u32, u32}[] [{6124107, 6124107}, {6124107, 6124107}] ("Colors [4]") cluster{u32, u32}[] [{6618880, 6618880}, {6618880, 6618880}] ("Colors [4]") cluster{u32, u32}[] [{16318208, 16318208}, {16318208, 16318208}] ("Colors [4]") cluster{u32, u32}[] [{8554752, 8554752}, {8554752, 8554752}] ("Colors [4]")] -> w648
                      tunnel: [FALSE FALSE FALSE TRUE] -> w647
                      frame Default {
                      }
                      frame "TEMPERATURE_STABILIZED" {
                      }
                      frame "TEMPERATURE_NOT_STABILIZED" {
                      }
                      frame "TEMPERATURE_NOT_REACHED" {
                      }
                    }
                    n264 = case shown="\"TEMPERATURE_NOT_REACHED\"" w645 {
                      tunnel: [cluster{u32, u32}[] [{6124107, 6124107}, {6124107, 6124107}] ("Colors [4]") cluster{u32, u32}[] [{6618880, 6618880}, {6618880, 6618880}] ("Colors [4]") cluster{u32, u32}[] [{16318208, 16318208}, {16318208, 16318208}] ("Colors [4]") cluster{u32, u32}[] [{8554752, 8554752}, {8554752, 8554752}] ("Colors [4]")] -> w644
                      tunnel: [FALSE FALSE FALSE TRUE] -> w643
                      frame Default {
                      }
                      frame "TEMPERATURE_STABILIZED" {
                      }
                      frame "TEMPERATURE_NOT_STABILIZED" {
                      }
                      frame "TEMPERATURE_NOT_REACHED" {
                      }
                    }
                    n265 = property on="Cooler status 1" class="Bool (strict)"("Colors [4]"=w653, "Blinking"=w652) -> ()  [unwired: 2 in, 2 out]
                    n266 = property class="Bool (strict)"("Colors [4]"=w653, "Blinking"=w652) -> ()  [unwired: 2 in, 2 out]
                    n267 = property on="Cooler status 4" class="Bool (strict)"("Colors [4]"=w644, "Blinking"=w643) -> ()  [unwired: 2 in, 2 out]
                    n268 = property on="Cooler status 3" class="Bool (strict)"("Colors [4]"=w648, "Blinking"=w647) -> ()  [unwired: 2 in, 2 out]
                    n269 = property on="Panel cooler 4" class="Bool (strict)"("Colors [4]"=w644, "Blinking"=w643) -> ()  [unwired: 2 in, 2 out]
                    n270 = property on="Cooler status 2" class="Bool (strict)"("Colors [4]"=w651, "Blinking"=w650) -> ()  [unwired: 2 in, 2 out]
                    n271 = property on="Panel cooler 3" class="Bool (strict)"("Colors [4]"=w648, "Blinking"=w647) -> ()  [unwired: 2 in, 2 out]
                    n272 = property on="Panel cooler 2" class="Bool (strict)"("Colors [4]"=w651, "Blinking"=w650) -> ()  [unwired: 2 in, 2 out]
                  }
                  frame #2 {
                    n273 = Unbundle By Name(w714) -> ("CamStatus"=w707:string, "connection"=w700:bool)
                    n274 = Unbundle By Name(w713) -> ("CamStatus"=w709:string, "connection"=w696:bool)
                    n275 = Unbundle By Name(w712) -> ("CamStatus"=w710:string, "connection"=w695:bool)
                    n276 = Unbundle By Name(w715) -> ("CamStatus"=w705:string, "connection"=w702:bool)
                    n277 = case shown="True" w695 {
                      tunnel: [u32 16739417 w721] -> w711
                      tunnel: w710 -> [_ w718]
                      tunnel: w704 -> [_ w719]
                      tunnel: ["" ("CamStatus") w718] -> w697
                      frame False {
                      }
                      frame True {
                        n278 = property on="Acq status string ch4" class="Str"() -> ("Text.BGColor"=w720:u32)  [unwired: 2 in, 2 out]
                        n279 = case shown="Default" w718 {
                          tunnel: [w724 u32 13882323 u32 13882323] -> w721
                          tunnel: w719 -> [w723 _ _]
                          tunnel: w720 -> [w722 _ _]
                          frame Default {
                            n280 = case shown="True" w723 {
                              tunnel: [w725 w729] -> w724
                              tunnel: w722 -> [w725 w726]
                              frame False {
                              }
                              frame True {
                                n281 = Equal?(x=w726, y=u32 16776002) -> (x = y?=w728:bool)
                                n282 = case shown="True" w728 {
                                tunnel: [u32 16776002 u32 9346816] -> w729
                                frame False {
                                }
                                frame True {
                                }
                                }
                              }
                            }
                          }
                          frame "IDLE" {
                          }
                          frame "" {
                            # "sem resposta do ACS"
                          }
                        }
                      }
                    }
                    "Acq status string ch4" <- w697
                    n283 = case shown="True" w702 {
                      tunnel: w705 -> [_ w772]
                      tunnel: w704 -> [_ w775]
                      tunnel: [u32 16739417 w773] -> w703
                      tunnel: ["" ("CamStatus") w772] -> w701
                      frame False {
                      }
                      frame True {
                        n284 = property on="Acq status string ch1" class="Str"() -> ("Text.BGColor"=w774:u32)  [unwired: 2 in, 2 out]
                        n285 = case shown="Default" w772 {
